vi "Bin Logging Message Loop.vi"(8 "error in (no error)":errorcluster, 10 "Data Queue":refnum<queue>, 11 "Message Queues":T1) -> (0 "error out":errorcluster)   [LabVIEW 2017, in "Logging.lvlib"]
uses:
  Logging.lvlib
  support/Message Queue/All Message Queues.ctl
  support/Message Queue/Message Cluster.ctl
  Logging Configuration.ctl
  Logging State.ctl
  support/Message Queue/Enqueue Message (Single).vi
  <vilib>/Utility/error.llb/Error Cluster From Error Code.vi
  <vilib>/ErrorRing/Error Ring.xnode
  support/Message Queue/Message Queue.lvlib
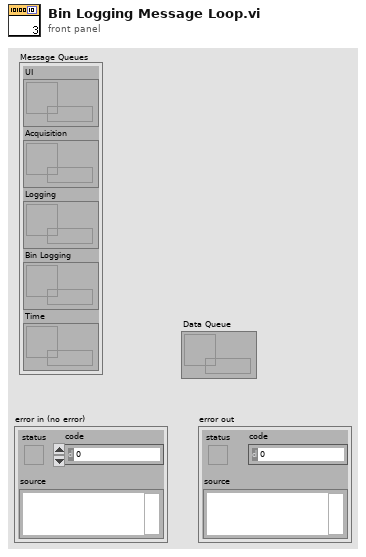
[diagram p1: front panel]
types:
  T1 = typedef "Message Queue.lvlib/All Message Queues.ctl" = cluster{"UI":refnum<queue>, "Acquisition":refnum<queue>, "Logging":refnum<queue>, "Bin Logging":refnum<queue>, "Time":refnum<queue>}
  T2 = typedef "Logging.lvlib/Logging Configuration.ctl" = cluster{"Log File Base Path":path, "TDMS File Reference":refnum<k34>, "Log File Offsite Path":path, "Project code":string, "Bin File Reference":refnum<file>}
  T3 = typedef "Logging.lvlib/Logging State.ctl" = enum16{"Idle", "Logging"}
  T4 = enum16{"open", "replace", "create", "open or create", "replace or create", "replace or create with confirmation"}
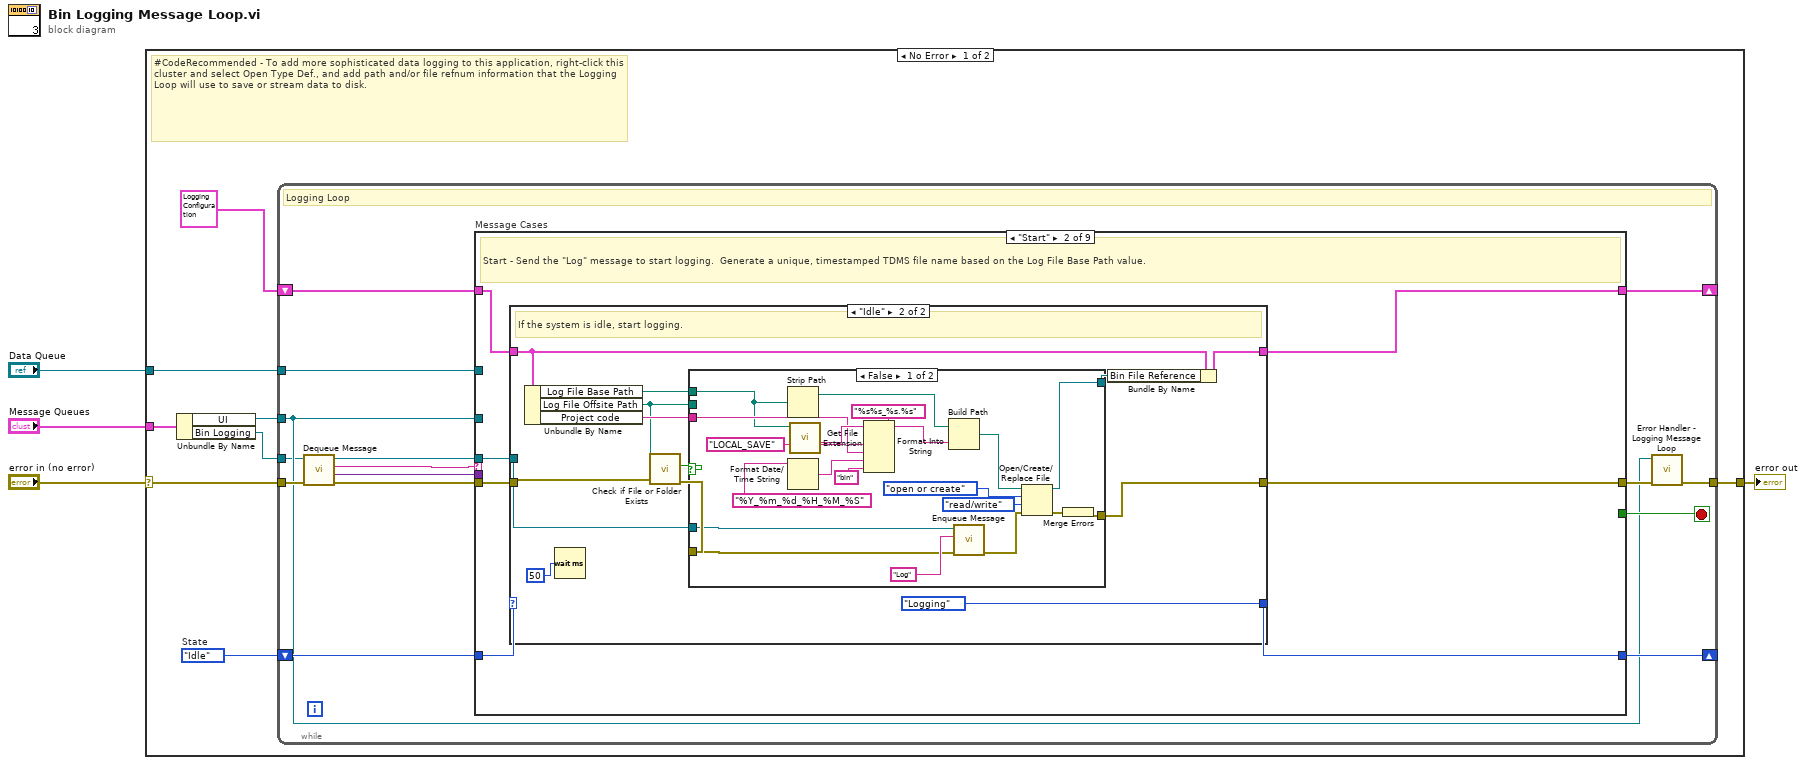
[diagram p0: block diagram]
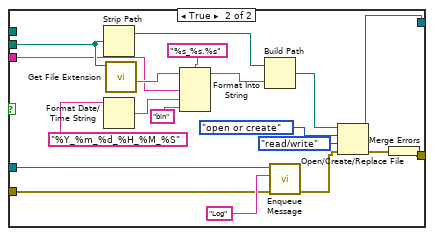
[diagram p4: hidden frame]
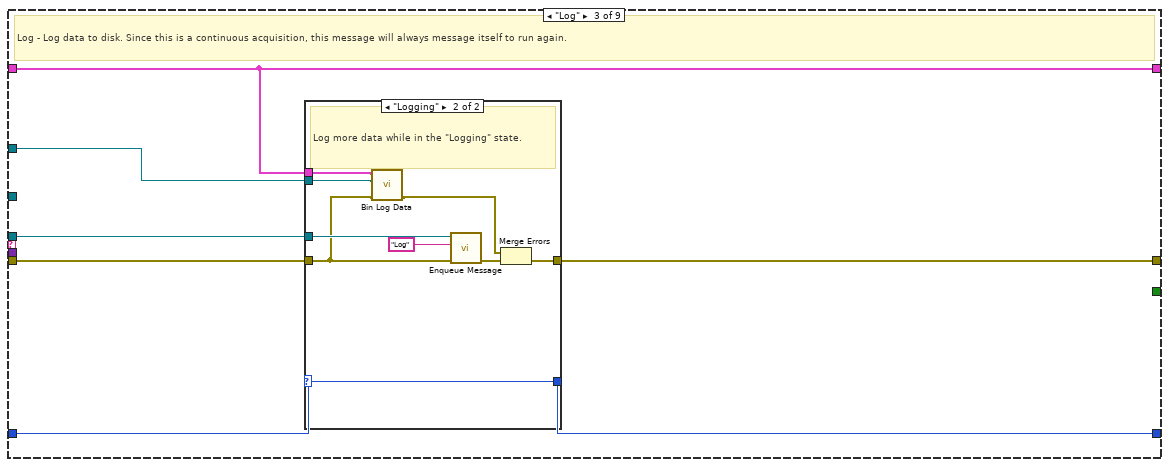
[diagram p5: hidden frame]
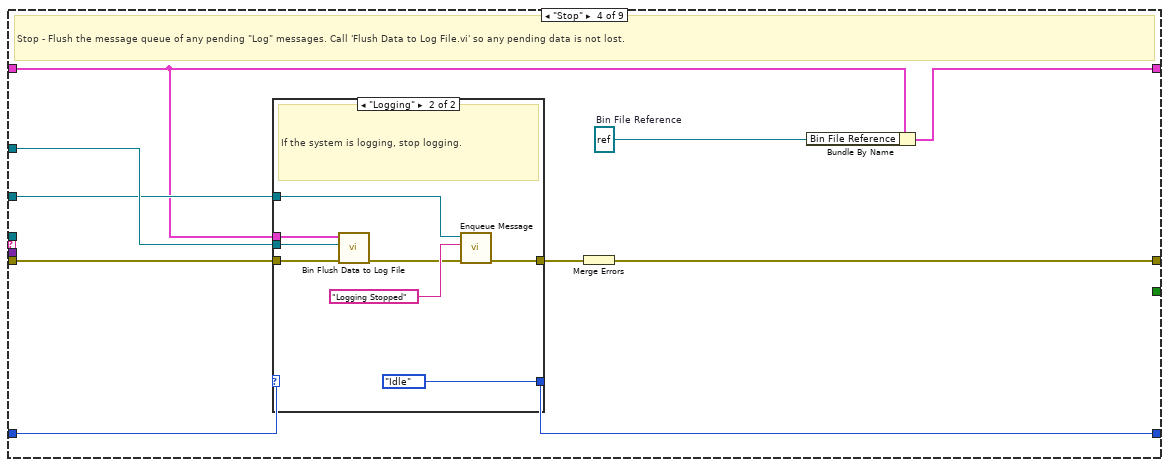
[diagram p7: hidden frame]
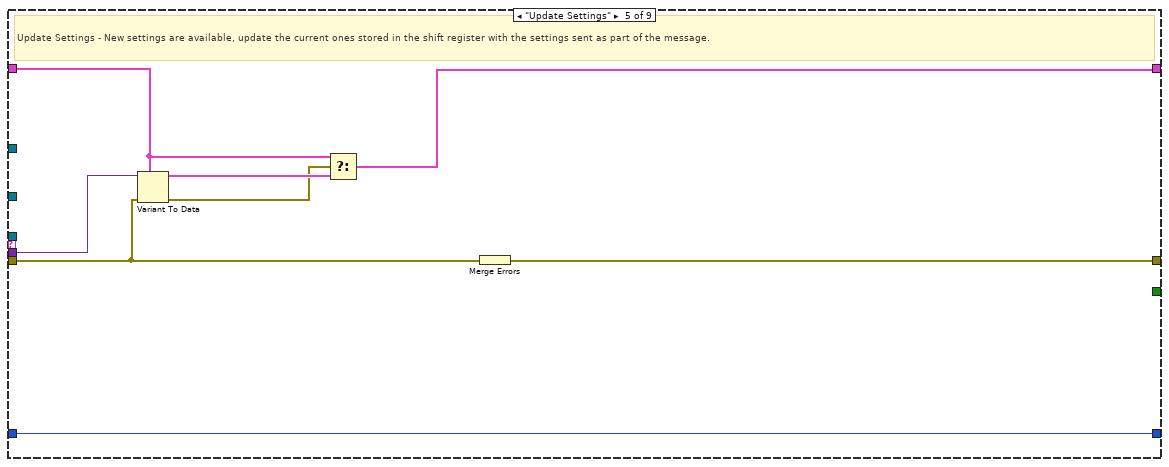
[diagram p9: hidden frame]
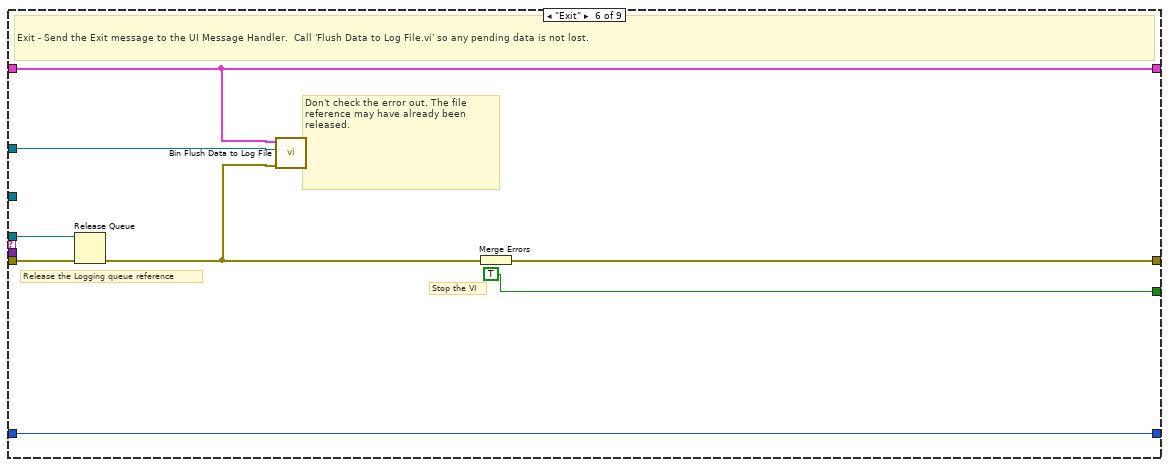
[diagram p10: hidden frame]
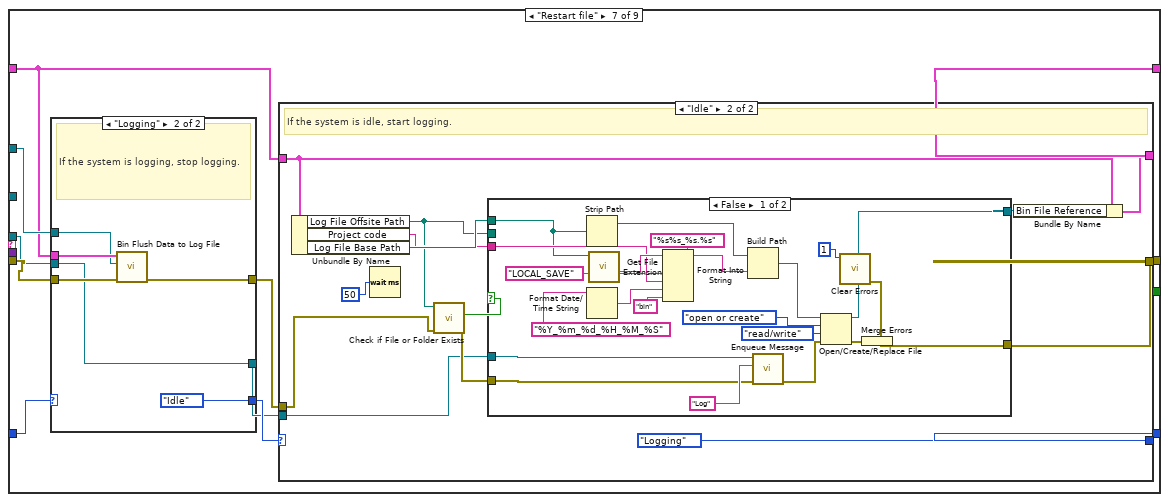
[diagram p11: hidden frame]
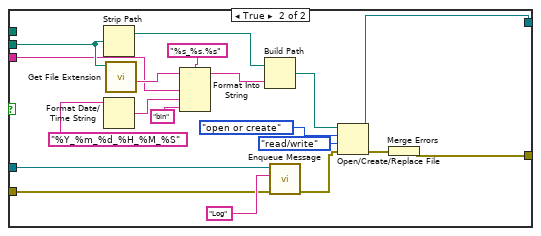
[diagram p13: hidden frame]
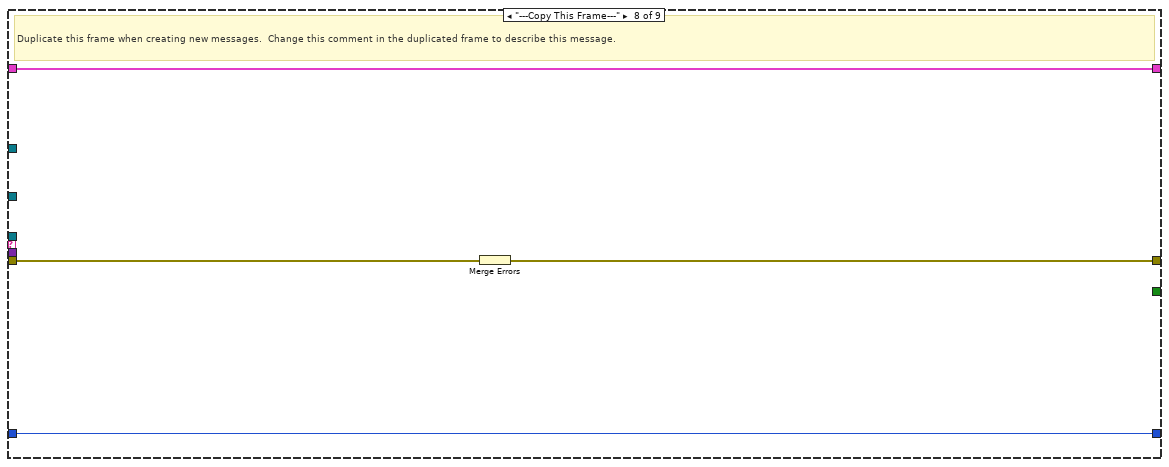
[diagram p15: hidden frame]
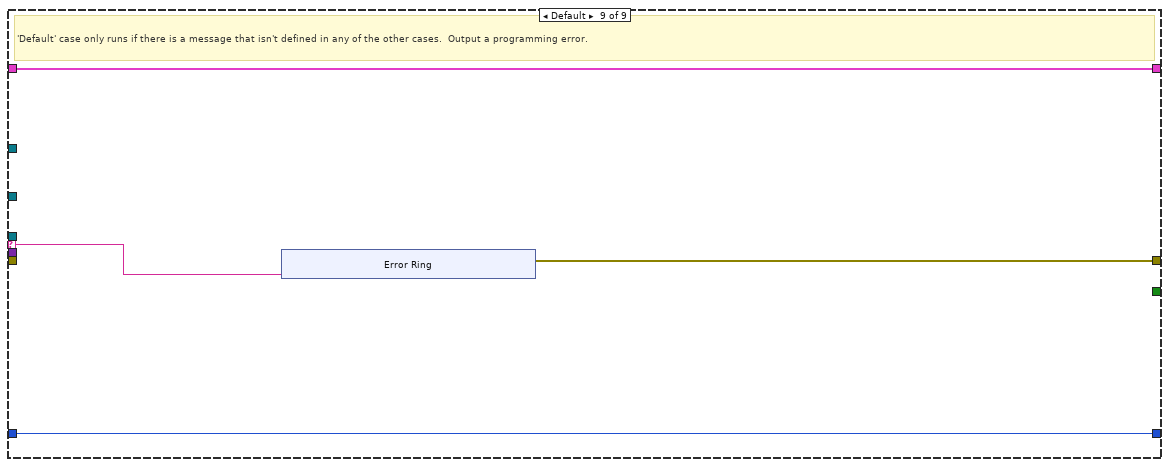
[diagram p16: hidden frame]
diagram:
  n1 = case shown="No Error" "error in (no error)" {
    selector: "error in (no error)" -> [w9 w235]
    tunnel: "Message Queues" -> [w12 _]
    tunnel: [w11 w235] -> w3
    tunnel: "Data Queue" -> [w8 _]
    frame No Error {
      w6 = Logging_State."Idle"  # State
      # "#CodeRecommended - To add more sophisticated data logging to this application, right-click this cluster and select Open Type Def., and add path and/or file refnum information that the Logging Loop will use to save or stream data to disk."
      n2 = Unbundle By Name(w12) -> ("UI"=w7:refnum<queue>, "Bin Logging"=w5:refnum<queue>)
      n3 = while {
        shift-right: [w27] -> _
        shift-left: T2 {"Log File Base Path"=path "", "TDMS File Reference"=refnum, "Log File Offsite Path"=path "", "Project code"="", "Bin File Reference"=refnum} ("Logging Configuration") -> [w14]
        tunnel: w7 -> [w16]
        tunnel: w8 -> [w21]
        shift-right: [w19] -> _
        shift-left: w6 -> [w20]
        tunnel: w9 -> [w25]
        tunnel: [w18] -> w11
        tunnel: w5 -> [w15]
        stop <- w26 stop-if-true
        # "Logging Loop"
        n4 = call "Dequeue Message.vi"("error in (no error)"=w25, "Message Queue"=w15) -> ("error out"=w24:errorcluster, "Message Data"=w23:variant, "Message"=w13:string, "dup Message Queue"=w22:refnum<queue>)  [unwired: 6 in]
        n5 = case "Message Cases" shown="\"Start\"" w13 {
          selector: w13 -> [_ _ _ _ _ _ _ _ w224]
          tunnel: w22 -> [_ w36 w97 _ _ w142 w155 _ _]
          tunnel: w24 -> [w29 w35 w95 w116 w130 w143 w156 w223 _]
          tunnel: [w29 w37 w98 w119 w137 w144 w151 w221 w225] -> w17
          tunnel: w14 -> [w30 w34 w94 w112 w136 w140 w146 w222 w227]
          tunnel: [w30 w33 w94 w111 w133 w140 w150 w222 w227] -> w27
          tunnel: [_ _ _ _ _ TRUE _ _ _] -> w26
          tunnel: w23 -> [_ _ _ _ w131 _ _ _ _]
          tunnel: w16 -> [_ _ _ w113 _ _ _ _ _]
          tunnel: w21 -> [_ _ w96 w117 _ w138 w148 _ _]
          tunnel: w20 -> [w28 w32 w93 w115 w132 w141 w149 w220 w226]
          tunnel: [w28 w31 w92 w114 w132 w141 w152 w220 w226] -> w19
          frame "Initialize" {
            # "Initialize - gets called when first launched. Currently a no-op."
          }
          frame "Start" {
            # "Start - Send the \"Log\" message to start logging.  Generate a unique, timestamped TDMS file name based on the Log File Base Path value."
            n6 = case shown="\"Idle\"" w32 {
              selector: w32 -> [w39 _]
              tunnel: [w38 w49] -> w37
              tunnel: w36 -> [_ w50]
              tunnel: w35 -> [w38 w41]
              tunnel: w34 -> [w40 w51]
              tunnel: [w40 w53] -> w33
              tunnel: [w39 Logging_State."Logging" ("State")] -> w31
              frame "Logging" {
                # "The system is already logging. Ignore the \"Start\" message."
              }
              frame "Idle" {
                # "If the system is idle, start logging."
                n7 = Unbundle By Name(w51) -> ("Log File Base Path"=w43:path, "Log File Offsite Path"=w46:path, "Project code"=w48:string)
                n8 = Wait (ms)(milliseconds to wait=u32 50) -> ()  [unwired: 1 out]
                n9 = call <vilib>:"Check if File or Folder Exists.vi"("error in (no error)"=w41, "path"=w46) -> ("error out"=w45:errorcluster, "file or folder exists?"=w44:bool)  [unwired: 7 in, 1 out]
                n10 = case shown="False" w44 {
                  tunnel: w46 -> [_ w90]
                  tunnel: w50 -> [w61 w82]
                  tunnel: [w60 w81] -> w49
                  tunnel: w48 -> [w57 w80]
                  tunnel: w45 -> [w62 w75]
                  tunnel: [w58 w74] -> w47
                  tunnel: w43 -> [w55 _]
                  frame False {
                    n11 = Strip Path(path=w55) -> (stripped path=w70:path)  [unwired: 1 out]
                    n12 = Format Date/Time String(time format string (%c)="%Y_%m_%d_%H_%M_%S") -> (date/time string=w68:string)  [unwired: 2 in]
                    n13 = call <vilib>:"Get File Extension.vi"("file"=w55) -> ("filename without extension"=w71:string)  [unwired: 6 in, 4 out]
                    n14 = Format Into String(format string="%s%s_%s.%s", initial string=w71, "LOCAL_SAVE" ("input 1"), w57, w68, "bin" ("input 3")) -> (resulting string=w66:string)  [unwired: 1 in, 1 out]
                    n15 = Build Path(base path=w70, name or relative path=w66) -> (appended path=w65:path)
                    n16 = call-poly "Enqueue Message.vi"("error in (no error)"=w62, "Message"="Log", "Message Queue"=w61) -> ("error out"=w54:errorcluster)  [unwired: 7 in, 1 out]
                    n17 = Open/Create/Replace File(file path (use dialog)=w65, error in=w54, operation (0:open)=T4."open or create", access (0:read/write)=enum16{"read/write", "read-only", "write-only"}."read/write") -> (refnum out=w58:refnum<file>, error out=w59:errorcluster)  [unwired: 2 in, 1 out]
                    n18 = Merge Errors(w59) -> (w60:errorcluster)
                  }
                  frame True {
                    n19 = Strip Path(path=w90) -> (stripped path=w87:path)  [unwired: 1 out]
                    n20 = Format Date/Time String(time format string (%c)="%Y_%m_%d_%H_%M_%S") -> (date/time string=w85:string)  [unwired: 2 in]
                    n21 = call <vilib>:"Get File Extension.vi"("file"=w90) -> ("filename without extension"=w88:string)  [unwired: 6 in, 4 out]
                    n22 = Format Into String(format string="%s_%s.%s", initial string=w88, w80, w85, "bin" ("input 3")) -> (resulting string=w83:string)  [unwired: 1 in, 1 out]
                    n23 = Build Path(base path=w87, name or relative path=w83) -> (appended path=w78:path)
                    n24 = call-poly "Enqueue Message.vi"("error in (no error)"=w75, "Message"="Log", "Message Queue"=w82) -> ()  [unwired: 7 in, 2 out]
                    n25 = Open/Create/Replace File(file path (use dialog)=w78, error in=w75, operation (0:open)=T4."open or create", access (0:read/write)=enum16{"read/write", "read-only", "write-only"}."read/write") -> (refnum out=w74:refnum<file>, error out=w79:errorcluster)  [unwired: 2 in, 1 out]
                    n26 = Merge Errors(w79) -> (w81:errorcluster)
                  }
                }
                n27 = Bundle By Name(cluster=w51, "Bin File Reference"=w47) -> (w53:T2)
              }
            }
          }
          frame "Log" {
            # "Log - Log data to disk. Since this is a continuous acquisition, this message will always message itself to run again."
            n28 = case shown="\"Logging\"" w93 {
              selector: w93 -> [w100 w105]
              tunnel: [w99 w109] -> w98
              tunnel: w97 -> [_ w107]
              tunnel: w96 -> [_ w103]
              tunnel: w95 -> [w99 w102]
              tunnel: w94 -> [_ w104]
              tunnel: [w100 w105] -> w92
              frame "Idle" {
                # "Ignore \"Log\" messages when the logging is idle."
              }
              frame "Logging" {
                # "Log more data while in the \"Logging\" state."
                n29 = call "Bin Log Data.vi"("error in (no error)"=w102, "Data Queue"=w103, "Logging Configuration"=w104) -> ("error out"=w101:errorcluster)  [unwired: 8 in]
                n30 = call-poly "Enqueue Message.vi"("error in (no error)"=w102, "Message"="Log", "Message Queue"=w107) -> ("error out"=w108:errorcluster)  [unwired: 7 in, 1 out]
                n31 = Merge Errors(w101, w108) -> (w109:errorcluster)
              }
            }
          }
          frame "Stop" {
            w110 = refnum<file> refnum  # Bin File Reference
            # "Stop - Flush the message queue of any pending \"Log\" messages. Call 'Flush Data to Log File.vi' so any pending data is not lost."
            n32 = case shown="\"Logging\"" w115 {
              selector: w115 -> [w120 _]
              tunnel: [w121 w128] -> w118
              tunnel: w117 -> [_ w124]
              tunnel: w112 -> [_ w125]
              tunnel: w116 -> [w121 w123]
              tunnel: [w120 Logging_State."Idle" ("State")] -> w114
              tunnel: w113 -> [_ w127]
              frame "Idle" {
                # "The system is already idle. Ignore the \"Stop\" message."
              }
              frame "Logging" {
                # "If the system is logging, stop logging."
                n33 = call "Bin Flush Data to Log File.vi"("error in (no error)"=w123, "Data Queue"=w124, "Logging Configuration"=w125) -> ("error out"=w122:errorcluster)  [unwired: 8 in]
                n34 = call-poly "Enqueue Message.vi"("error in (no error)"=w122, "Message"="Logging Stopped", "Message Queue"=w127) -> ("error out"=w128:errorcluster)  [unwired: 7 in, 1 out]
              }
            }
            n35 = Merge Errors(w118) -> (w119:errorcluster)
            n36 = Bundle By Name(cluster=w112, "Bin File Reference"=w110) -> (w111:T2)
          }
          frame "Update Settings" {
            # "Update Settings - New settings are available, update the current ones stored in the shift register with the settings sent as part of the message."
            n37 = Variant To Data(error in=w130, type=w136, Variant=w131) -> (data=w135:T2, error out=w134:errorcluster)
            n38 = Select(t=w136, s=w134, f=w135) -> (s? t:f=w133:T2)
            n39 = Merge Errors(w130) -> (w137:errorcluster)
          }
          frame "Exit" {
            # "Don't check the error out. The file reference may have already been released."
            # "Release the Logging queue reference"
            # "Stop the VI"
            # "Exit - Send the Exit message to the UI Message Handler.  Call 'Flush Data to Log File.vi' so any pending data is not lost."
            n40 = Release Queue(queue=w142, error in (no error)=w143) -> (error out=w139:errorcluster)  [unwired: 1 in, 2 out]
            n41 = call "Bin Flush Data to Log File.vi"("error in (no error)"=w139, "Data Queue"=w138, "Logging Configuration"=w140) -> ()  [unwired: 8 in, 1 out]
            n42 = Merge Errors(w139) -> (w144:errorcluster)
          }
          frame "Restart file" {
            n43 = case shown="\"Logging\"" w149 {
              selector: w149 -> [w212 _]
              tunnel: [w213 w216] -> w154
              tunnel: w155 -> [_ w214]
              tunnel: w146 -> [_ w218]
              tunnel: w156 -> [w213 w217]
              tunnel: [w212 Logging_State."Idle" ("State")] -> w153
              tunnel: w148 -> [_ w215]
              tunnel: [_ w214] -> w147
              frame "Idle" {
                # "The system is already idle. Ignore the \"Stop\" message."
              }
              frame "Logging" {
                # "If the system is logging, stop logging."
                n44 = call "Bin Flush Data to Log File.vi"("error in (no error)"=w217, "Data Queue"=w215, "Logging Configuration"=w218) -> ("error out"=w216:errorcluster)  [unwired: 8 in]
              }
            }
            n45 = case shown="\"Idle\"" w153 {
              selector: w153 -> [w159 _]
              tunnel: [w158 w171] -> w151
              tunnel: [w157 w162] -> w150
              tunnel: [w159 Logging_State."Logging" ("State")] -> w152
              tunnel: w146 -> [w157 w163]
              tunnel: w154 -> [w158 w160]
              tunnel: w147 -> [_ w165]
              frame "Logging" {
                # "The system is already logging. Ignore the \"Start\" message."
              }
              frame "Idle" {
                # "If the system is idle, start logging."
                n46 = Unbundle By Name(w163) -> ("Log File Offsite Path"=w166:path, "Project code"=w167:string, "Log File Base Path"=w168:path)
                n47 = Wait (ms)(milliseconds to wait=u32 50) -> ()  [unwired: 1 out]
                n48 = call <vilib>:"Check if File or Folder Exists.vi"("error in (no error)"=w160, "path"=w166) -> ("error out"=w169:errorcluster, "file or folder exists?"=w170:bool)  [unwired: 7 in, 1 out]
                n49 = case shown="False" w170 {
                  tunnel: w166 -> [_ w210]
                  tunnel: w165 -> [w181 w202]
                  tunnel: [w180 w201] -> _
                  tunnel: w167 -> [w176 w200]
                  tunnel: w169 -> [w182 w195]
                  tunnel: [w177 w194] -> w164
                  tunnel: w168 -> [w174 _]
                  frame False {
                    n50 = Strip Path(path=w174) -> (stripped path=w190:path)  [unwired: 1 out]
                    n51 = Format Date/Time String(time format string (%c)="%Y_%m_%d_%H_%M_%S") -> (date/time string=w188:string)  [unwired: 2 in]
                    n52 = call <vilib>:"Get File Extension.vi"("file"=w174) -> ("filename without extension"=w191:string)  [unwired: 6 in, 4 out]
                    n53 = Format Into String(format string="%s%s_%s.%s", initial string=w191, "LOCAL_SAVE" ("input 1"), w176, w188, "bin" ("input 3")) -> (resulting string=w186:string)  [unwired: 1 in, 1 out]
                    n54 = Build Path(base path=w190, name or relative path=w186) -> (appended path=w185:path)
                    n55 = call-poly "Enqueue Message.vi"("error in (no error)"=w182, "Message"="Log", "Message Queue"=w181) -> ("error out"=w178:errorcluster)  [unwired: 7 in, 1 out]
                    n56 = Open/Create/Replace File(file path (use dialog)=w185, error in=w178, operation (0:open)=T4."open or create", access (0:read/write)=enum16{"read/write", "read-only", "write-only"}."read/write") -> (refnum out=w177:refnum<file>, error out=w179:errorcluster)  [unwired: 2 in, 1 out]
                    n57 = Merge Errors(w179) -> (w180:errorcluster)
                  }
                  frame True {
                    n58 = Strip Path(path=w210) -> (stripped path=w207:path)  [unwired: 1 out]
                    n59 = Format Date/Time String(time format string (%c)="%Y_%m_%d_%H_%M_%S") -> (date/time string=w205:string)  [unwired: 2 in]
                    n60 = call <vilib>:"Get File Extension.vi"("file"=w210) -> ("filename without extension"=w208:string)  [unwired: 6 in, 4 out]
                    n61 = Format Into String(format string="%s_%s.%s", initial string=w208, w200, w205, "bin" ("input 3")) -> (resulting string=w203:string)  [unwired: 1 in, 1 out]
                    n62 = Build Path(base path=w207, name or relative path=w203) -> (appended path=w198:path)
                    n63 = call-poly "Enqueue Message.vi"("error in (no error)"=w195, "Message"="Log", "Message Queue"=w202) -> ()  [unwired: 7 in, 2 out]
                    n64 = Open/Create/Replace File(file path (use dialog)=w198, error in=w195, operation (0:open)=T4."open or create", access (0:read/write)=enum16{"read/write", "read-only", "write-only"}."read/write") -> (refnum out=w194:refnum<file>, error out=w199:errorcluster)  [unwired: 2 in, 1 out]
                    n65 = Merge Errors(w199) -> (w201:errorcluster)
                  }
                }
                n66 = call <vilib>:"Clear Errors.vi"("specific error code to clear (0: all)"=1) -> ("error out"=w171:errorcluster)  [unwired: 5 in, 1 out]
                n67 = Bundle By Name(cluster=w163, "Bin File Reference"=w164) -> (w162:T2)
              }
            }
          }
          frame "---Copy This Frame---" {
            # "Duplicate this frame when creating new messages.  Change this comment in the duplicated frame to describe this message."
            n68 = Merge Errors(w223) -> (w221:errorcluster)
          }
          frame Default {
            # "'Default' case only runs if there is a message that isn't defined in any of the other cases.  Output a programming error."
            n69 = xnode "Error Ring"("parameter 0"=w224) -> ("error out"=w225:errorcluster)
          }
        }
        n70 = call "Error Handler - Logging Message Loop.vi"("error in (no error)"=w17, "Message Queue"=w16) -> ("dup error in"=w18:errorcluster)  [unwired: 8 in, 1 out]
      }
    }
    frame Error {
    }
  }
  "error out" <- w3
